vi "Write Test Suite Result.vi"(8 "error in (no error)":errorcluster, 10 "Test Suite Result":refnum<user-event>, 11 "Test Assert Factory in":refnum<class "Test Assert Factory.lvclass">) -> (0 "error out":errorcluster, 3 "Test Assert Factory out":refnum<class "Test Assert Factory.lvclass">)   [LabVIEW 2013, in "Caraya.lvlib" / "Test Assert Factory.lvclass"]
uses:
  Test Assert Factory.lvclass
  Test Result/Test Result.lvclass
  Test Assert Factory.lvclass/Test Assert Factory.ctl
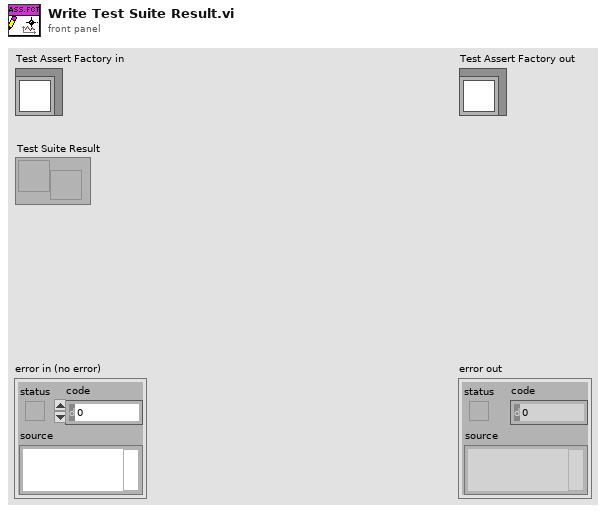
[diagram p1: front panel]
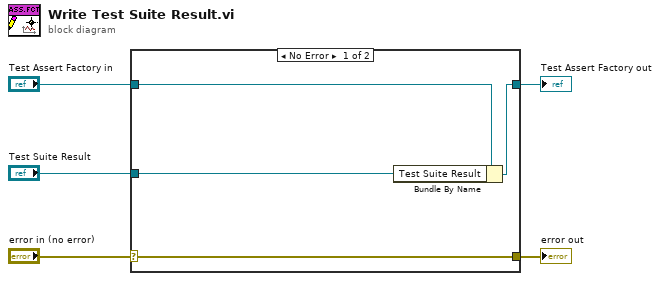
[diagram p0: block diagram]
diagram:
  n1 = case shown="No Error" "error in (no error)" {
    selector: "error in (no error)" -> [w9 w10]
    tunnel: [w9 w10] -> w4
    tunnel: [w7 w11] -> w2
    tunnel: "Test Assert Factory in" -> [w8 w11]
    tunnel: "Test Suite Result" -> [w6 _]
    frame No Error {
      n2 = Bundle By Name(cluster=w8, "Test Suite Result"=w6) -> (w7:refnum<class "Test Assert Factory.lvclass">)
    }
    frame Error {
    }
  }
  "error out" <- w4
  "Test Assert Factory out" <- w2
